vi "PassThru.Do.vi"(8 "error in (no error)":errorcluster, 10 "State Variables":T1, 11 "gRPC Request":T13) -> (0 "error out":errorcluster, 2 "State Variables out":T1, 3 "gRPC Response":T15)   [LabVIEW 2025, in "bus_monitor_server_do.lvlib"]
uses:
  bus_monitor_server_do.lvlib
  Types/MainProcess.StateVariables.ctl
  Types/XNET.InitialSettings.ctl
  bus_monitor_server/RPC Messages/ni_bus_monitor_api_ConnectSettings.ctl
  bus_monitor_server/RPC Messages/ni_bus_monitor_api_CanMode.ctl
  bus_monitor_server/RPC Messages/ni_bus_monitor_api_Termination.ctl
  bus_monitor_server/RPC Messages/ni_bus_monitor_api_FdIsoMode.ctl
  bus_monitor_server/RPC Messages/ni_bus_monitor_api_FilterInfo.ctl
  bus_monitor_server/RPC Messages/ni_bus_monitor_api_DirectionFilter.ctl
  bus_monitor_server/RPC Messages/ni_bus_monitor_api_FrameFilter.ctl
  Types/StreamProcess.Refs.ctl
  Types/StreamProcess.VIRef.ctl
  bus_monitor_server/RPC Messages/ni_bus_monitor_api_Session.ctl
  bus_monitor_server/RPC Messages/ni_bus_monitor_api_PassThruReply.ctl
  bus_monitor_server/RPC Messages/ni_bus_monitor_api_ErrorInfo.ctl
  bus_monitor_server/RPC Messages/ni_bus_monitor_api_PassThruRequest.ctl
  bus_monitor_server/RPC Messages/ni_bus_monitor_api_Frame.ctl
  <vilib>/xnet/xnet.llb/XNET Frame CAN.ctl
  <vilib>/xnet/xnet.llb/XNET Frame Type CAN.ctl
  <vilib>/xnet/xnet.llb/XNET Write (Frame CAN).vi
  bus_monitor_server/bus_monitor_server.lvlib
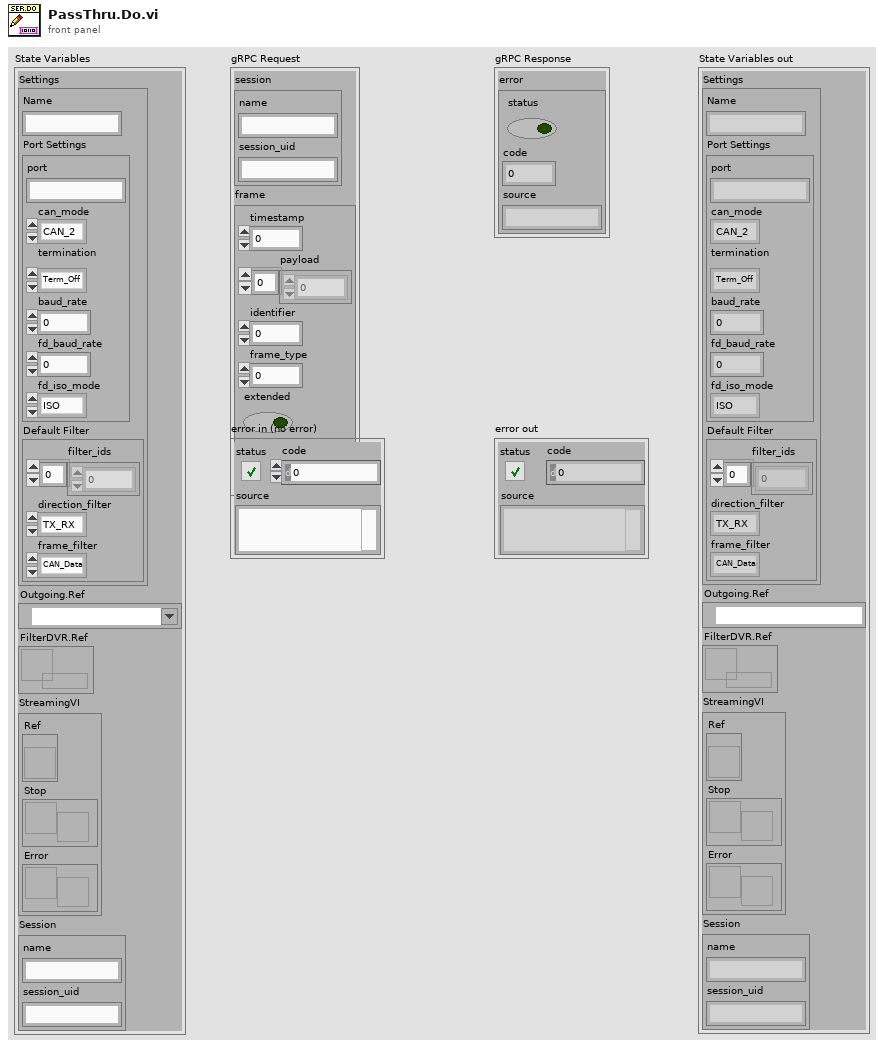
[diagram p1: front panel]
types:
  T1 = typedef "bus_monitor_server_do.lvlib/MainProcess.StateVariables.ctl" = cluster{"Settings":T2, "Outgoing.Ref":refnum<k21>, "FilterDVR.Ref":refnum<data-value>, "StreamingVI":T10, "Session":T12}
  T2 = typedef "bus_monitor_server_do.lvlib/XNET.InitialSettings.ctl" = cluster{"Name":string, "Port Settings":T3, "Default Filter":T7}
  T3 = typedef "bus_monitor_server.lvlib/ni_bus_monitor_api_ConnectSettings.ctl" = cluster{"port":string, "can_mode":T4, "termination":T5, "baud_rate":u64, "fd_baud_rate":u64, "fd_iso_mode":T6}
  T4 = typedef "bus_monitor_server.lvlib/ni_bus_monitor_api_CanMode.ctl" = enum32{"CAN_2", "CAN_FD", "CAN_FD_BRS"}
  T5 = typedef "bus_monitor_server.lvlib/ni_bus_monitor_api_Termination.ctl" = enum32{"Term_Off", "Term_On"}
  T6 = typedef "bus_monitor_server.lvlib/ni_bus_monitor_api_FdIsoMode.ctl" = enum32{"ISO", "Non_ISO", "ISO_Legacy"}
  T7 = typedef "bus_monitor_server.lvlib/ni_bus_monitor_api_FilterInfo.ctl" = cluster{"filter_ids":u32[], "direction_filter":T8, "frame_filter":T9}
  T8 = typedef "bus_monitor_server.lvlib/ni_bus_monitor_api_DirectionFilter.ctl" = enum32{"TX_RX", "RX", "TX"}
  T9 = typedef "bus_monitor_server.lvlib/ni_bus_monitor_api_FrameFilter.ctl" = enum32{"CAN_Data", "CAN_Remote", "CAN_Bus_Error", "CAN_2_Data", "CAN_FD_Data", "CAN_FD_BRS_Data", "J1939_Data", "Delay", "Log_Trigger", "Start_Trigger", "All"}
  T10 = typedef "bus_monitor_server_do.lvlib/StreamProcess.Refs.ctl" = cluster{"Ref":T11, "Stop":refnum<notifier>, "Error":refnum<notifier>}
  T11 = typedef "bus_monitor_server_do.lvlib/StreamProcess.VIRef.ctl" = refnum<vi>
  T12 = typedef "bus_monitor_server.lvlib/ni_bus_monitor_api_Session.ctl" = cluster{"name":string, "session_uid":string}
  T13 = typedef "bus_monitor_server.lvlib/ni_bus_monitor_api_PassThruRequest.ctl" = cluster{"session":T12, "frame":T14}
  T14 = typedef "bus_monitor_server.lvlib/ni_bus_monitor_api_Frame.ctl" = cluster{"timestamp":dbl, "payload":u8[], "identifier":u32, "frame_type":u32, "extended":bool, "echo":bool}
  T15 = typedef "bus_monitor_server.lvlib/ni_bus_monitor_api_PassThruReply.ctl" = cluster{"error":T16}
  T16 = typedef "bus_monitor_server.lvlib/ni_bus_monitor_api_ErrorInfo.ctl" = errorcluster
  T17 = typedef "XNET Frame CAN.ctl" = cluster{"timestamp":timestamp, "payload":u8[], "identifier":u32, "type":T18, "extended?":bool, "echo?":bool}
  T18 = typedef "XNET Frame Type CAN.ctl" = u8
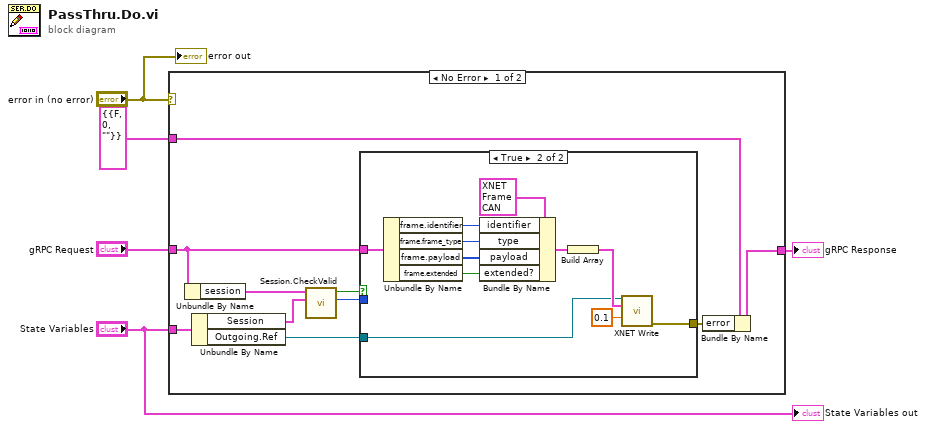
[diagram p0: block diagram]
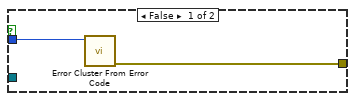
[diagram p2: hidden frame]
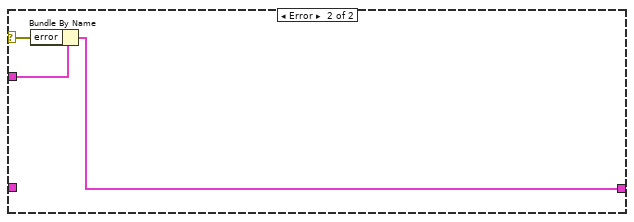
[diagram p3: hidden frame]
diagram:
  n1 = case shown="No Error" "error in (no error)" {
    selector: "error in (no error)" -> [_ w30]
    tunnel: [w14 w29] -> w5
    tunnel: "gRPC Request" -> [w11 _]
    tunnel: "State Variables" -> [w13 _]
    tunnel: T15 {"error"={"status"=FALSE, "code"=0, "source"=""}} ("Message Data") -> [w12 w31]
    frame No Error {
      n2 = Unbundle By Name(w11) -> ("session"=w8:T12)
      n3 = Unbundle By Name(w13) -> ("Session"=w9:T12, "Outgoing.Ref"=w10:refnum<k21>)
      n4 = call "Session.CheckValid.vi"("Cached Session"=w9, "requested session"=w8) -> ("Error Code"=w6:i32, "Valid?"=w7:bool)  [unwired: 8 in]
      n5 = case shown="True" w7 {
        tunnel: w11 -> [_ w21]
        tunnel: [w17 w19] -> w15
        tunnel: w10 -> [_ w18]
        tunnel: w6 -> [w16 _]
        frame False {
          n6 = call <vilib>:"Error Cluster From Error Code.vi"("error code (0)"=w16) -> ("error out"=w17:errorcluster)  [unwired: 8 in]
        }
        frame True {
          n7 = Unbundle By Name(w21) -> ("frame.identifier"=w25:u32, "frame.frame_type"=w24:u32, "frame.payload"=w23:u8[], "frame.extended"=w22:bool)
          n8 = Bundle By Name(cluster=T17 {"timestamp"=timestamp(0 s since 1904-01-01), "payload"=[], "identifier"=0, "type"=0, "extended?"=FALSE, "echo?"=FALSE} ("CAN frame"), "identifier"=w25, "type"=w24, "payload"=w23, "extended?"=w22) -> (w27:T17)
          n9 = Build Array(w27) -> (w20:T17[])
          n10 = call-poly <vilib>:"XNET Write.vi"("session in"=w18, "data"=w20, "timeout (10)"=0.1) -> ("error out"=w19:errorcluster)  [unwired: 11 in, 1 out]
        }
      }
      n11 = Bundle By Name(cluster=w12, "error"=w15) -> (w14:T15)
    }
    frame Error {
      n12 = Bundle By Name(cluster=w31, "error"=w30) -> (w29:T15)
    }
  }
  "gRPC Response" <- w5
  "State Variables out" <- "State Variables"
  "error out" <- "error in (no error)"
